vi "Set Limits.vi"(0 "VISA Session":refnum<visa-resource-name>="GPIB0::6::INSTR", 5 "Model In":string="KLP", 7 "channel name (\"1\")":string="\"1\"", 9 "Raw Model In":string="KLR", 11 "error in (no error)":errorcluster) -> (4 "VISA Session Out":refnum<visa-resource-name>="GPIB0::6::INSTR", 6 "Model Out":string="KLP", 8 "channel name out (\"\")":string="\"1\"" caption="channel name Out (\"\")", 10 "Max Current Limit":dbl=32.0 caption="Max Current" format="%^.2e", 12 "Min Voltage Limit":dbl caption="Min Voltage" format="%^.2e", 13 "Max Voltage Limit":dbl=75.0 caption="Max Voltage" format="%^.2e", 14 "Min Current Limit":dbl=0.37 caption="Min Current" format="%^.2e", 15 "error out":errorcluster)   [LabVIEW 2013]
doc: "Used to establish limits for Kepco power supplies.\nValid for KLP and KLR , BOP 1000W, BHK prodcuts only\nRaw model required connection required for KLP product.\n\nModel in used to determine if product requires password to access limit configuration. (KLP and KLR)\nRAW model in - allows for KLP verse KLR differences (limits verses virtual model.\n\nFunction is not meant for standalone opearation as visa open and close is not present in fucntion."
panel:
  out "Instrument Error":errorcluster
  in  "Return":bool
  in  "Set Limits":bool
  in  "Enable Password":bool
  in  "Voltage Limit":dbl=75.0 format="%^.2e"
  in  "Current Limit":dbl=32.0 format="%^.2e"
  in  "Password":string
  # "SETTING LIMITS"
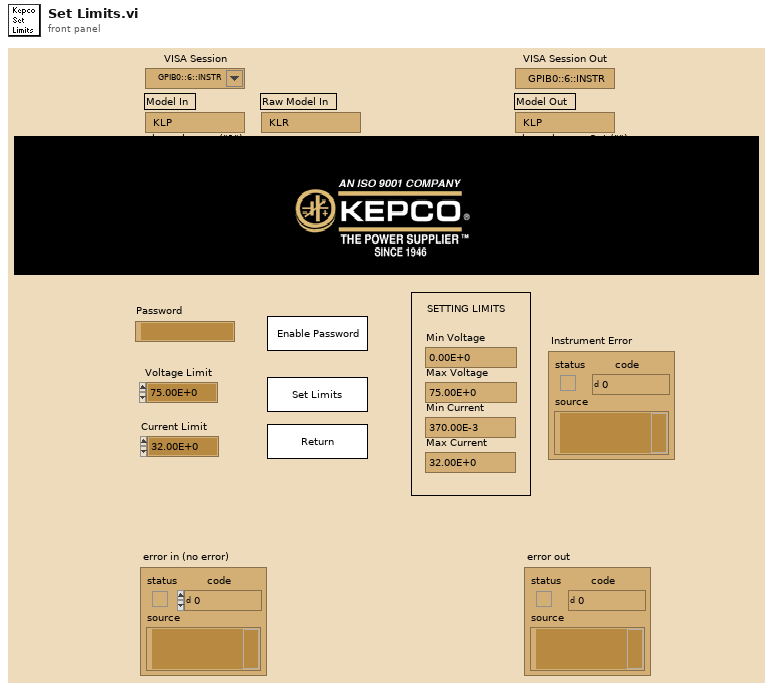
[diagram p1: front panel]
types:
  T1 = cluster{bool, "error code":i32, "error message":string}
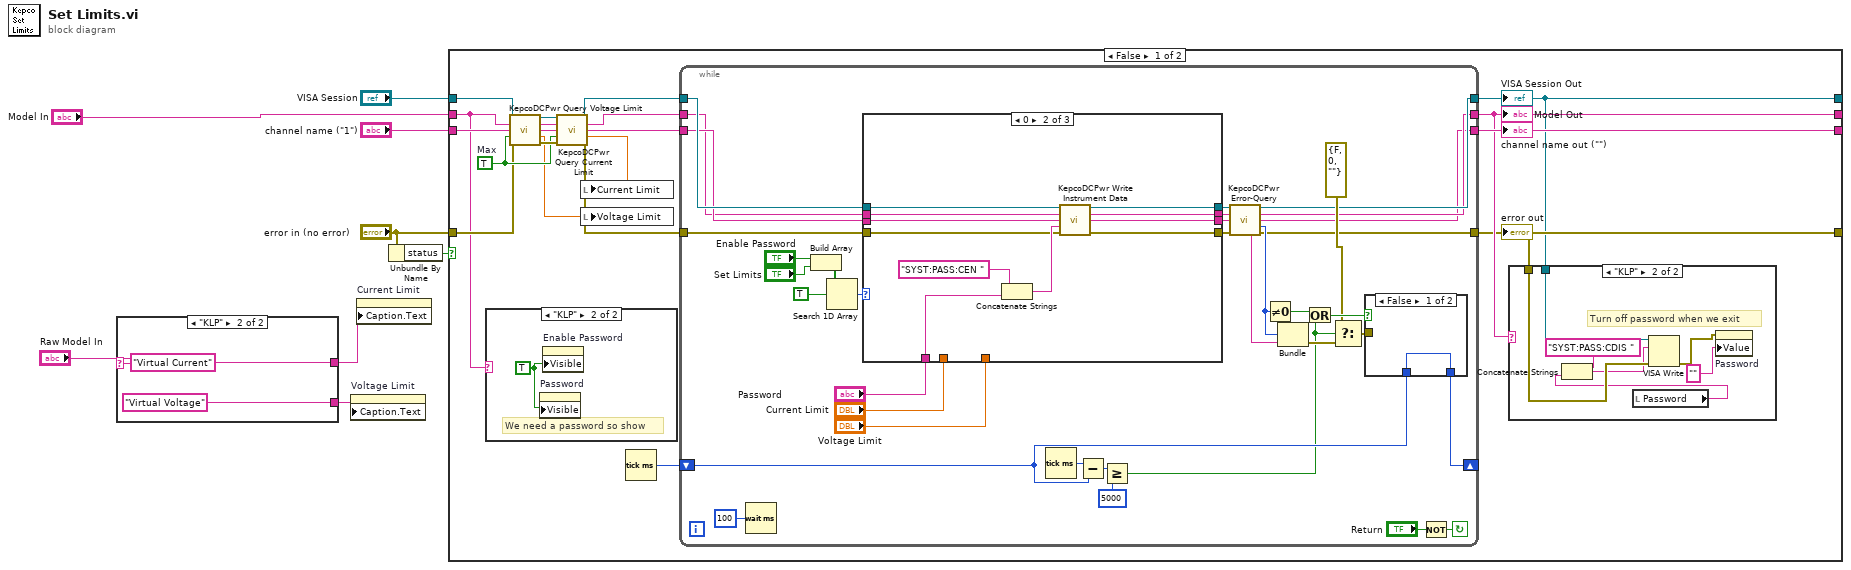
[diagram p0: block diagram]
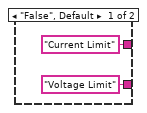
[diagram p2: hidden frame]
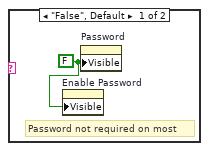
[diagram p4: hidden frame]
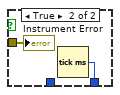
[diagram p5: hidden frame]
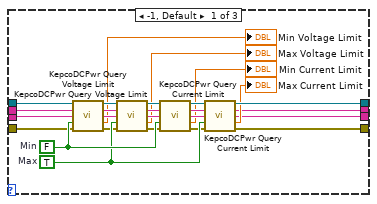
[diagram p6: hidden frame]
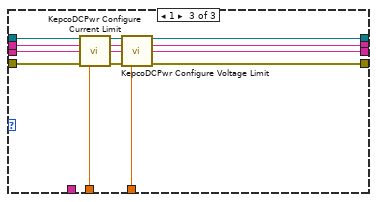
[diagram p7: hidden frame]
diagram:
  n1 = case shown="\"KLP\"" "Raw Model In" {
    tunnel: ["Current Limit" ("Label.Text") "Virtual Current" ("Label.Text")] -> w4
    tunnel: ["Voltage Limit" ("Unit Label.Text") "Virtual Voltage" ("Unit Label.Text")] -> w3
    frame "False", Default {
    }
    frame "KLP" {
    }
  }
  n2 = property on="Voltage Limit" class="DigNum (strict)"("Caption.Text"=w3) -> ()  [unwired: 2 in, 2 out]
  n3 = property on="Current Limit" class="DigNum (strict)"("Caption.Text"=w4) -> ()  [unwired: 2 in, 2 out]
  n4 = Unbundle By Name("error in (no error)") -> ("status"=w12:bool)
  n5 = case shown="False" w12 {
    tunnel: "error in (no error)" -> [w25 w136]
    tunnel: "VISA Session" -> [w30 w139]
    tunnel: "Model In" -> [w20 w138]
    tunnel: "channel name (\"1\")" -> [w28 w137]
    tunnel: [w18 w139] -> w8
    tunnel: [w19 w138] -> w7
    tunnel: [w36 w137] -> w6
    tunnel: [w17 w136] -> w1
    frame False {
      w31 = TRUE  # Max
      n6 = case shown="\"KLP\"" w20 {
        frame "False", Default {
          w44 = FALSE ("Visible")
          # "Password not required on most"
          n7 = property on="Enable Password" class="Bool"("Visible"=w44) -> ()  [unwired: 2 in, 2 out]
          n8 = property on="Password" class="Str"("Visible"=w44) -> ()  [unwired: 2 in, 2 out]
        }
        frame "KLP" {
          w45 = TRUE ("Visible")
          # "We need a password so show"
          n9 = property on="Password" class="Str"("Visible"=w45) -> ()  [unwired: 2 in, 2 out]
          n10 = property on="Enable Password" class="Bool"("Visible"=w45) -> ()  [unwired: 2 in, 2 out]
        }
      }
      n11 = call "KepcoDCPwr Query Voltage Limit.vi"("VISA Session"=w30, "Model In"=w20, "channel name (\"\")"=w28, "Max Level (T),MIN LEVEL(F)"=w31, "error in (no error)"=w25) -> ("VISA Session Out"=w35:refnum<visa-resource-name>, "Model Out"=w33:string, "channel name out (\"\")"=w32:string, "voltage level"=w22:dbl, "error out"=w34:errorcluster)  [unwired: 6 out]
      n12 = call "KepcoDCPwr Query Current Limit.vi"("VISA Session"=w35, "Model In"=w33, "channel name (\"\")"=w32, "Level"=w31, "error in (no error)"=w34) -> ("VISA Session Out"=w29:refnum<visa-resource-name>, "Model Out"=w26:string, "channel name out (\"\")"=w27:string, "current limit"=w23:dbl, "error out"=w24:errorcluster)  [unwired: 6 out]
      n13 = local write "Current Limit"(w23) -> ()
      n14 = local write "Voltage Limit"(w22) -> ()
      n15 = Tick Count (ms)() -> (millisecond timer value=w21:u32)
      n16 = while {
        shift-left: w21 -> [w48]
        shift-right: [w47] -> _
        tunnel: w24 -> [w81]
        tunnel: [w54] -> w17
        tunnel: [w52] -> w36
        tunnel: [w53] -> w19
        tunnel: [w55] -> w18
        tunnel: w27 -> [w79]
        tunnel: w26 -> [w78]
        tunnel: w29 -> [w80]
        stop <- w71 continue-if-true
        n17 = Wait (ms)(milliseconds to wait=u32 100) -> ()  [unwired: 1 out]
        n18 = Build Array("Enable Password", "Set Limits") -> (w75:bool[])
        n19 = Search 1D Array(1D array=w75, element=TRUE) -> (index of element=w73:i32)  [unwired: 1 in]
        n20 = case shown="0" w73 {
          tunnel: w81 -> [w97 w112 w135]
          tunnel: w80 -> [w96 w119 w133]
          tunnel: [w92 w118 w132] -> w56
          tunnel: w79 -> [w93 w116 w130]
          tunnel: w78 -> [w94 w117 w128]
          tunnel: "Current Limit" -> [_ _ w127]
          tunnel: "Voltage Limit" -> [_ _ w126]
          tunnel: "Password" -> [_ w111 _]
          tunnel: [w87 w115 w131] -> w51
          tunnel: [w86 w114 w129] -> w50
          tunnel: [w85 w113 w134] -> w49
          frame -1, Default {
            w105 = FALSE  # Min
            w104 = TRUE  # Max
            n21 = call "KepcoDCPwr Query Voltage Limit.vi"("VISA Session"=w96, "Model In"=w94, "channel name (\"\")"=w93, "Max Level (T),MIN LEVEL(F)"=w105, "error in (no error)"=w97) -> ("VISA Session Out"=w106:refnum<visa-resource-name>, "Model Out"=w99:string, "channel name out (\"\")"=w109:string, "voltage level"=→"Min Voltage Limit":dbl, "error out"=w98:errorcluster)  [unwired: 6 out]
            n22 = call "KepcoDCPwr Query Voltage Limit.vi"("VISA Session"=w106, "Model In"=w99, "channel name (\"\")"=w109, "Max Level (T),MIN LEVEL(F)"=w104, "error in (no error)"=w98) -> ("VISA Session Out"=w107:refnum<visa-resource-name>, "Model Out"=w103:string, "channel name out (\"\")"=w110:string, "voltage level"=→"Max Voltage Limit":dbl, "error out"=w100:errorcluster)  [unwired: 6 out]
            n23 = call "KepcoDCPwr Query Current Limit.vi"("VISA Session"=w107, "Model In"=w103, "channel name (\"\")"=w110, "Level"=w105, "error in (no error)"=w100) -> ("VISA Session Out"=w108:refnum<visa-resource-name>, "Model Out"=w102:string, "channel name out (\"\")"=w95:string, "current limit"=→"Min Current Limit":dbl, "error out"=w101:errorcluster)  [unwired: 6 out]
            n24 = call "KepcoDCPwr Query Current Limit.vi"("VISA Session"=w108, "Model In"=w102, "channel name (\"\")"=w95, "Level"=w104, "error in (no error)"=w101) -> ("VISA Session Out"=w92:refnum<visa-resource-name>, "Model Out"=w87:string, "channel name out (\"\")"=w86:string, "current limit"=→"Max Current Limit":dbl, "error out"=w85:errorcluster)  [unwired: 6 out]
          }
          frame 0 {
            n25 = Concatenate Strings("SYST:PASS:CEN ", w111) -> (w121:string)
            n26 = call "KepcoDCPwr Write Instrument Data.vi"("VISA Session"=w119, "Model"=w117, "channel name (\"\")"=w116, "Write Buffer"=w121, "error in (no error)"=w112) -> ("VISA Session Out"=w118:refnum<visa-resource-name>, "Model Out"=w115:string, "channel name out (\"\")"=w114:string, "error out"=w113:errorcluster)  [unwired: 7 out]
          }
          frame 1 {
            n27 = call "KepcoDCPwr Configure Current Limit.vi"("VISA Session"=w133, "Model In"=w128, "channel name (\"\")"=w130, "error in (no error)"=w135, "limit (0.0)"=w127) -> ("VISA Session Out"=w125:refnum<visa-resource-name>, "Model Out"=w123:string, "channel name out (\"\")"=w122:string, "error out"=w124:errorcluster)  [unwired: 7 out]
            n28 = call "KepcoDCPwr Configure Voltage Limit.vi"("VISA Session"=w125, "Model In"=w123, "channel name (\"\")"=w122, "error in (no error)"=w124, "limit (0.0)"=w126) -> ("VISA Session Out"=w132:refnum<visa-resource-name>, "Model Out"=w131:string, "channel name out (\"\")"=w129:string, "error out"=w134:errorcluster)  [unwired: 7 out]
          }
        }
        n29 = Tick Count (ms)() -> (millisecond timer value=w66:u32)
        n30 = Subtract(x=w66, y=w48) -> (x-y=w65:u32)
        n31 = Greater Or Equal?(x=w65, y=u32 5000) -> (x >= y?=w46:bool)
        n32 = call "KepcoDCPwr Error-Query.vi"("VISA Session"=w56, "Model In"=w51, "channel name (\"\")"=w50, "error in (no error)"=w49) -> ("VISA Session Out"=w55:refnum<visa-resource-name>, "Model Out"=w53:string, "channel name out (\"\")"=w52:string, "error code"=w61:i32, "error message"=w62:string, "error out"=w54:errorcluster)  [unwired: 6 out]
        n33 = Not Equal To 0?(x=w61) -> (x != 0?=w60:bool)
        n34 = Bundle(w60, "error code"=w61, "error message"=w62) -> (w59:T1)  [unwired: 1 out]
        n35 = Or(x=w60, y=w46) -> (x .or. y?=w63:bool)
        n36 = Select(t=T1 {FALSE, "error code"=0, "error message"=""}, s=w46, f=w59) -> (s? t:f=w58:T1)
        n37 = case shown="False" w63 {
          tunnel: [w82 w84] -> w47
          tunnel: w48 -> [w82 _]
          tunnel: w58 -> [_ w83]
          frame False {
          }
          frame True {
            n38 = Tick Count (ms)() -> (millisecond timer value=w84:u32)
            "Instrument Error" <- w83
          }
        }
        n39 = Not(x="Return") -> (.not. x?=w71:bool)
      }
      n40 = case shown="\"KLP\"" w19 {
        tunnel: w18 -> [_ w43]
        tunnel: w17 -> [_ w42]
        frame "False", Default {
        }
        frame "KLP" {
          # "Turn off password when we exit"
          n41 = local read "Password"() -> (w40:string)
          n42 = Concatenate Strings("SYST:PASS:CDIS " ("write buffer"), w40) -> (w39:string)
          n43 = VISA Write(VISA resource name=w43, write buffer=w39, error in (no error)=w42) -> (error out=w37:errorcluster)  [unwired: 2 out]
          n44 = property on="Password" class="Str"(error in=w37, "Value"="" ("Password")) -> ()  [unwired: 1 in, 2 out]
        }
      }
    }
    frame True {
    }
  }
  "error out" <- w1
  "VISA Session Out" <- w8
  "Model Out" <- w7
  "channel name out (\"\")" <- w6
